vi "Mark Document Dirty.vi"(8 "error in (no error)":errorcluster, 11 "Plugin Session in":refnum<class "Plugin Session.lvclass">) -> (0 "error out":errorcluster, 3 "Plugin Session out":refnum<class "Plugin Session.lvclass">)   [LabVIEW 2021, in "CIF_InstrumentStudio Plugin SDK.lvlib" / "Plugin Session.lvclass"]
uses:
  Plugin Session.lvclass
  Plugin Session.lvclass/Plugin Session.ctl
  Read Session Id.vi
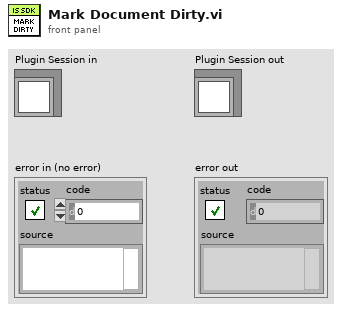
[diagram p1: front panel]
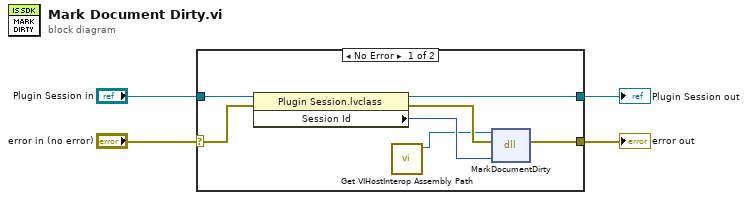
[diagram p0: block diagram]
diagram:
  n1 = case shown="No Error" "error in (no error)" {
    selector: "error in (no error)" -> [w9 w12]
    tunnel: "Plugin Session in" -> [w11 w13]
    tunnel: [w10 w13] -> w3
    tunnel: [w6 w12] -> w1
    frame No Error {
      n2 = property class="Plugin Session.lvclass"(reference=w11, error in=w9) -> (reference out=w10:refnum<class "Plugin Session.lvclass">, error out=w8:errorcluster, "Session Id"=w7:u64)
      n3 = call "Get VIHostInterop Assembly Path.vi"() -> ("VIHost.Interop Assembly"=w5:path)  [unwired: 11 in]
      n4 = dll-call lib="C:/ASW/Source/InstrumentStudio/IFDistribution/VIHostPanel/objects/export/targets/win64U/x64/msvc-14.0/debug/NationalInstruments.VIHost.Interop.dll" fn="MarkDocumentDirty"(path in=w5, error in=w8, "sessionId"=w7) -> (error out=w6:errorcluster)  [unwired: 3 in, 1 out]
    }
    frame Error {
    }
  }
  "Plugin Session out" <- w3
  "error out" <- w1
